vi "Get SMO Port.vi"(8 "error in (no error)":errorcluster, 11 "ExampleInstrument in":refnum<class "Instrument.Template.lvclass">) -> (0 "error out":errorcluster, 2 "Port":u16, 3 "ExampleInstrument out":refnum<class "Instrument.Template.lvclass">)   [LabVIEW 2019, in "Instrument.Template.lvclass"]
uses:
  Instrument.Template.lvclass
  Instrument Types/VSource/Instrument.VSource.lvclass
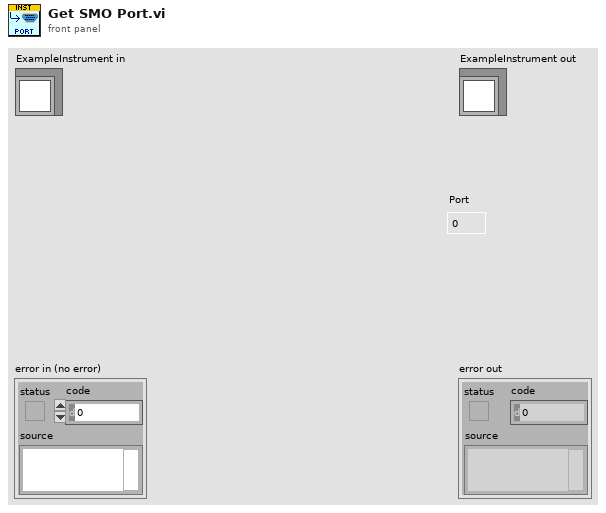
[diagram p1: front panel]
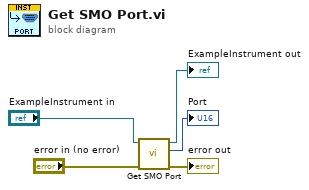
[diagram p0: block diagram]
diagram:
  n1 = call-parent "Get SMO Port.vi"("error in (no error)"="error in (no error)", "Instrument in"="ExampleInstrument in") -> ("error out"=→"error out":errorcluster, "Port"=→"Port":u16, "Instrument out"=→"ExampleInstrument out":refnum<class "Instrument.Template.lvclass">)  [unwired: 7 in]
